vi "Open_Create_CSV_File.vi"(0 "File Path Control":path, 11 "Error In":errorcluster) -> (4 "refnum out":refnum<file>, 6 "File Path":path, 15 "Error Out":errorcluster)   [LabVIEW 2021]
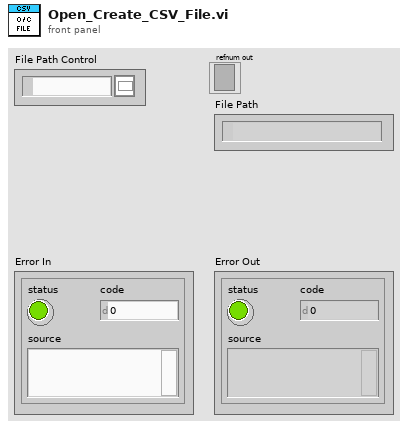
[diagram p1: front panel]
types:
  T1 = enum16{"open", "replace", "create", "open or create", "replace or create", "replace or create with confirmation"}
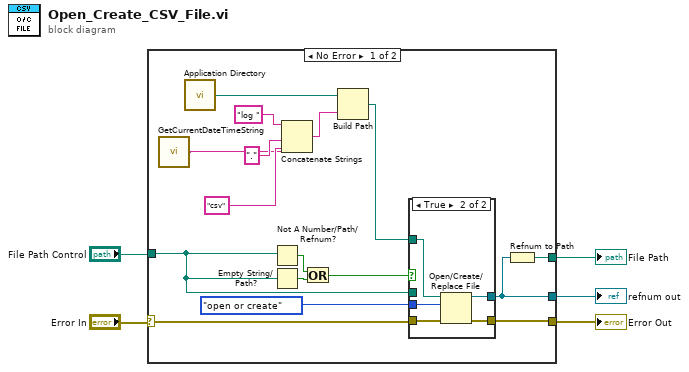
[diagram p0: block diagram]
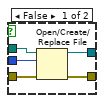
[diagram p2: hidden frame]
diagram:
  n1 = case shown="No Error" "Error In" {
    selector: "Error In" -> [w17 w32]
    tunnel: "File Path Control" -> [w15 _]
    tunnel: [w14 _] -> w4
    tunnel: [w16 w32] -> w2
    tunnel: [w13 _] -> w1
    frame No Error {
      n2 = call "GetCurrentDateTimeString.vi"() -> ("Date/Time String"=w6:string)  [unwired: 14 in, 1 out]
      n3 = call <vilib>:"Application Directory.vi"() -> ("Application Directory"=w12:path)
      n4 = Not A Number/Path/Refnum?(number/path/refnum=w15) -> (NaN/Path/Refnum?=w21:bool)
      n5 = Empty String/Path?(string/path=w15) -> (empty?=w20:bool)
      n6 = Concatenate Strings("log " ("string"), w6, "." ("string"), "csv") -> (w11:string)
      n7 = Or(x=w21, y=w20) -> (x .or. y?=w19:bool)
      n8 = Build Path(base path=w12, name or relative path=w11) -> (appended path=w9:path)
      n9 = case shown="True" w19 {
        tunnel: T1."open or create" ("operation (0:open)") -> [w24 w31]
        tunnel: [w25 w30] -> w14
        tunnel: w15 -> [w26 _]
        tunnel: w17 -> [w23 w29]
        tunnel: [w22 w28] -> w16
        tunnel: w9 -> [_ w27]
        frame False {
          n10 = Open/Create/Replace File(file path (use dialog)=w26, error in=w23, operation (0:open)=w24) -> (refnum out=w25:refnum<file>, error out=w22:errorcluster)  [unwired: 3 in, 1 out]
        }
        frame True {
          n11 = Open/Create/Replace File(file path (use dialog)=w27, error in=w29, operation (0:open)=w31) -> (refnum out=w30:refnum<file>, error out=w28:errorcluster)  [unwired: 3 in, 1 out]
        }
      }
      n12 = Refnum to Path(1:w14) -> (0:w13:path)
    }
    frame Error {
    }
  }
  "Error Out" <- w2
  "refnum out" <- w4
  "File Path" <- w1
